vi "RealImage_Create.vi"(8 "Error In":errorcluster, 10 "FileName":string, 11 "reference in":refnum<class "RealImage.lvclass">) -> (0 "Error Out":errorcluster, 3 "reference out":refnum<class "RealImage.lvclass">)   [LabVIEW 2020, in "RealImage.lvclass"]
uses:
  RealImage.lvclass
  RealImage.lvclass/RealImage.ctl
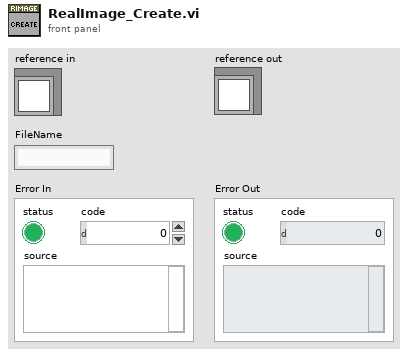
[diagram p1: front panel]
types:
  T1 = typedef "RealImage.lvclass/ObjectAttributes.ctl" = cluster{"_fileName":string}
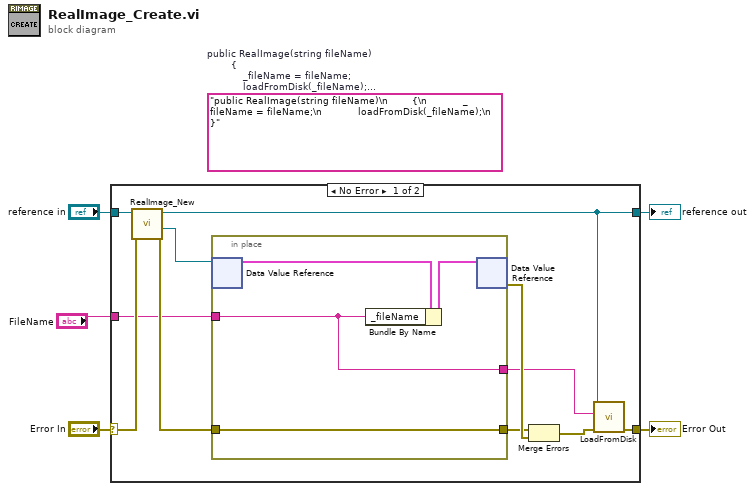
[diagram p0: block diagram]
diagram:
  (unwired) "public RealImage(string fileName)\n        {\n            _fileName = fileName;\n            loadFromDisk(_fileName);\n        }"  # public RealImage(string fileName)         {             _fileName = fileName;             loadFromDisk(_fileName);         }
  n1 = case shown="No Error" "Error In" {
    selector: "Error In" -> [w15 w22]
    tunnel: [w8 w22] -> w4
    tunnel: "reference in" -> [w16 w21]
    tunnel: [w7 w21] -> w2
    tunnel: "FileName" -> [w9 _]
    frame No Error {
      n2 = call "RealImage_New.vi"("error in (no error)"=w15, "reference in"=w16) -> ("error out"=w12:errorcluster, "DVRRefOut"=w13:refnum<data-value>, "reference out"=w7:refnum<class "RealImage.lvclass">)  [unwired: 6 in, 1 out]
      n3 = in-place {
        in-place-border: w12 -> [w18]
        in-place-border: [w18] -> w11
        in-place-border: w9 -> [w17]
        in-place-border: [w17] -> w6
        n4 = in-place-dvr #1(w13) -> (w19:T1)  [unwired: 1 out]
        n5 = Bundle By Name(cluster=w19, "_fileName"=w17) -> (w20:T1)
        n6 = in-place-dvr #1(w20) -> (w14:errorcluster)  [unwired: 1 out]
      }
      n7 = Merge Errors(w11, w14) -> (w10:errorcluster)
      n8 = call "LoadFromDisk.vi"("Error In"=w10, "FileName"=w6, "reference in"=w7) -> ("Error Out"=w8:errorcluster)  [unwired: 7 in, 1 out]
    }
    frame Error {
      # "VI-TechBaseTemplate_Simple_4x4x4"
    }
  }
  "Error Out" <- w4
  "reference out" <- w2
